vi "Galil_QR_single.vi"() -> ()   [LabVIEW 2011]
panel:
  in  "Galil.IGalil":refnum<k7>
  out "source":string="TIME"
  out "Number of Elements\nin Data Record":i32
  out "Description":string
  out "Units":string
  out "Sources":string[](array[string])
  out "sourceValue":dbl
  out "error out":errorcluster
  out "Connected To:":string
  in  "Connection String:":string
  # "This vi shows how to access data record information using the QR method with the Galil Communications Library.  \n\nIf Connection String is left blank, the vi will open the connections dialog when run.  If a value is input into Connection String, the vi will attempt to connect to the controller at that address (ie COM1 19200).\n\nThis vi gets all of the sources from the controller, and displays them into the Sources array.\nThen gets a data record and displays the value for TIME out of that data record"
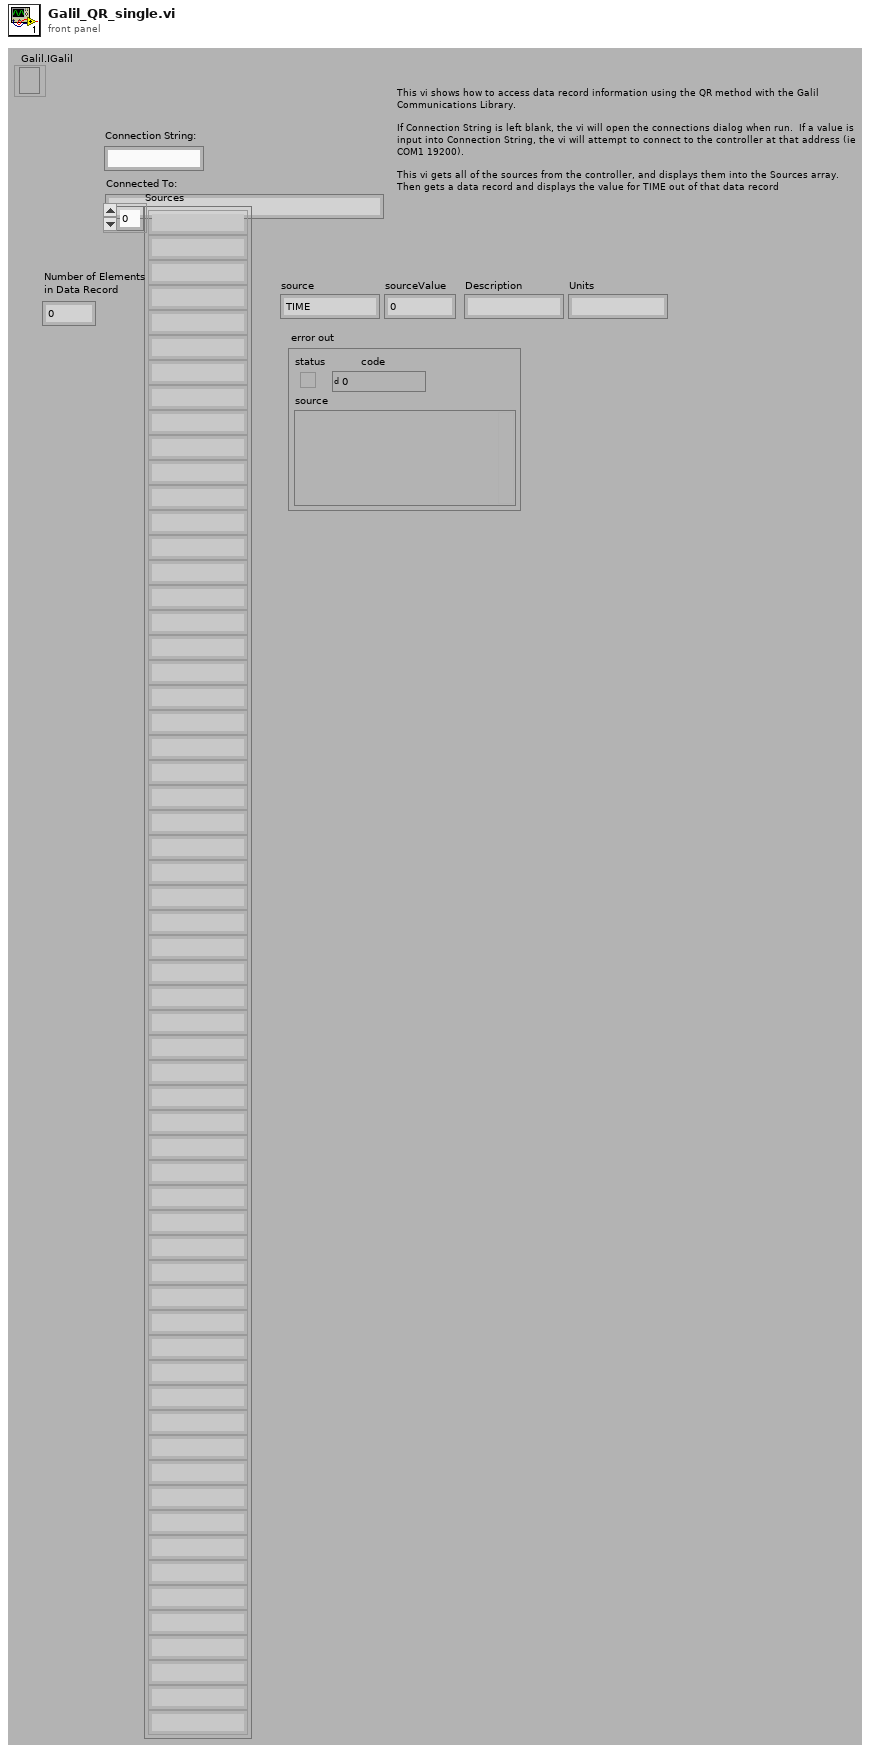
[diagram p1: front panel]
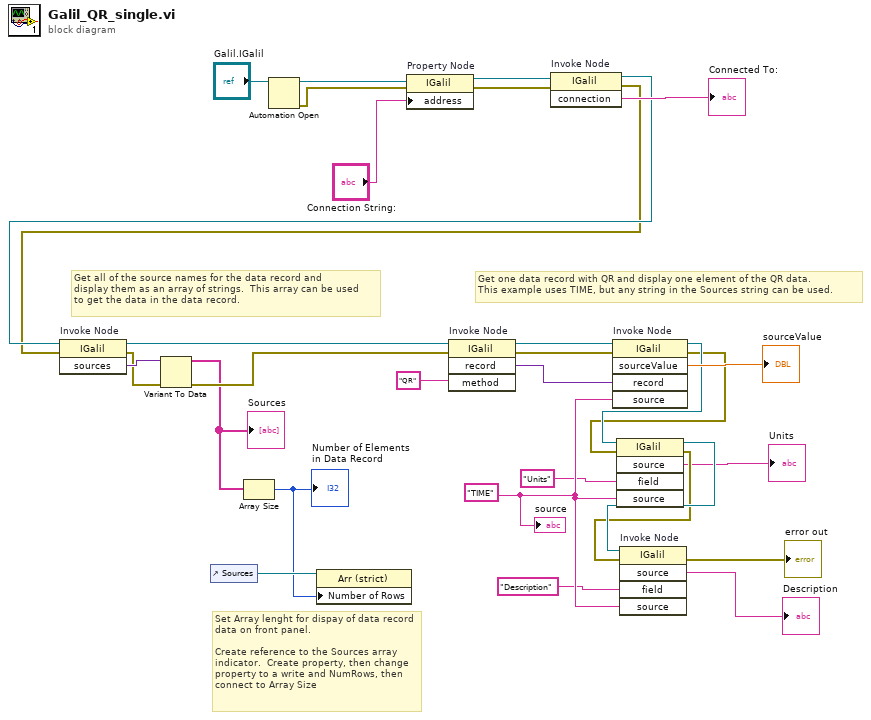
[diagram p0: block diagram]
diagram:
  w5 = "TIME"
  # "Set Array lenght for dispay of data record \ndata on front panel.\n\nCreate reference to the Sources array indicator.  Create property, then change property to a write and NumRows, then connect to Array Size"
  # "Get all of the source names for the data record and \ndisplay them as an array of strings.  This array can be used\nto get the data in the data record."
  # "Get one data record with QR and display one element of the QR data.  \nThis example uses TIME, but any string in the Sources string can be used."
  n1 = control-ref of="Sources"() -> (w11:refnum<vi>)
  n2 = Automation Open(Automation Refnum="Galil.IGalil") -> (Automation Refnum=w31:refnum<k7>, error out=w29:errorcluster)  [unwired: 1 in, 2 out]
  n3 = property on="Property Node" class="IGalil"(reference=w31, error in=w29, "address"="Connection String:") -> (reference out=w30:refnum<k7>, error out=w28:errorcluster)
  n4 = invoke on="Invoke Node" class="IGalil" method="connection"(reference=w30, error in=w28) -> (reference out=w23:refnum<k7>, error out=w21:errorcluster, "connection"=→"Connected To:":string)  [unwired: 1 in]
  n5 = invoke on="Invoke Node" class="IGalil" method="sources"(reference=w23, error in=w21) -> (reference out=w22:refnum<k7>, error out=w19:errorcluster, "sources"=w20:variant)  [unwired: 1 in]
  n6 = Variant To Data(error in=w19, Variant=w20) -> (data=w13:string[], error out=w18:errorcluster)  [unwired: 1 in]
  "Sources" <- w13
  n7 = Array Size(array=w13) -> (size(s)=w10:i32)
  "Number of Elements\nin Data Record" <- w10
  n8 = property class="Arr (strict)"(reference=w11, "Number of Rows"=w10) -> ()  [unwired: 1 in, 2 out]
  n9 = invoke on="Invoke Node" class="IGalil" method="record"(reference=w22, error in=w18, "method"="QR") -> (reference out=w17:refnum<k7>, error out=w16:errorcluster, "record"=w14:variant)  [unwired: 1 in, 1 out]
  n10 = invoke on="Invoke Node" class="IGalil" method="sourceValue"(reference=w17, error in=w16, "record"=w14, "source"=w5) -> (reference out=w8:refnum<k7>, error out=w7:errorcluster, "sourceValue"=→"sourceValue":dbl)  [unwired: 1 in, 2 out]
  n11 = invoke class="IGalil" method="source"(reference=w8, error in=w7, "field"="Units", "source"=w5) -> (reference out=w9:refnum<k7>, error out=w6:errorcluster, "source"=→"Units":string)  [unwired: 1 in, 2 out]
  n12 = invoke on="Invoke Node" class="IGalil" method="source"(reference=w9, error in=w6, "field"="Description", "source"=w5) -> (error out=→"error out":errorcluster, "source"=→"Description":string)  [unwired: 1 in, 3 out]
  "source" <- w5
